vi "Convert Data.vi"(8 "error in (no error)":errorcluster, 10 "Data In":refnum<class "Data.lvclass">, 11 "Converter in":refnum<class "Converter.lvclass">) -> (0 "error out":errorcluster, 2 "Data Out":refnum<class "Data.lvclass">, 3 "Converter out":refnum<class "Converter.lvclass">)   [LabVIEW 2022 SP3, in "Converter.lvclass"]
uses:
  Converter.lvclass
  Data/Data.lvclass
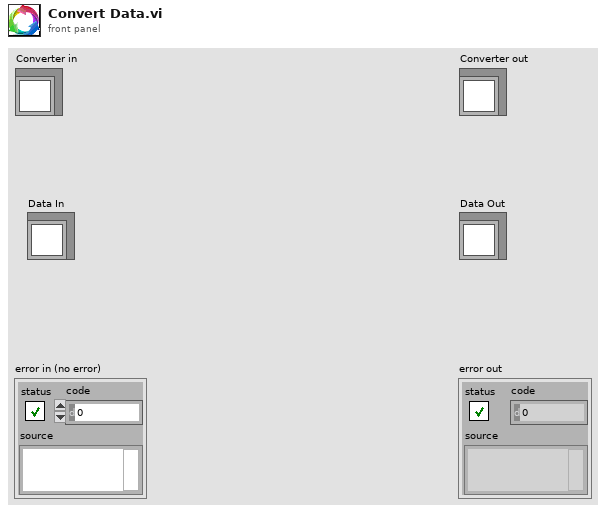
[diagram p1: front panel]
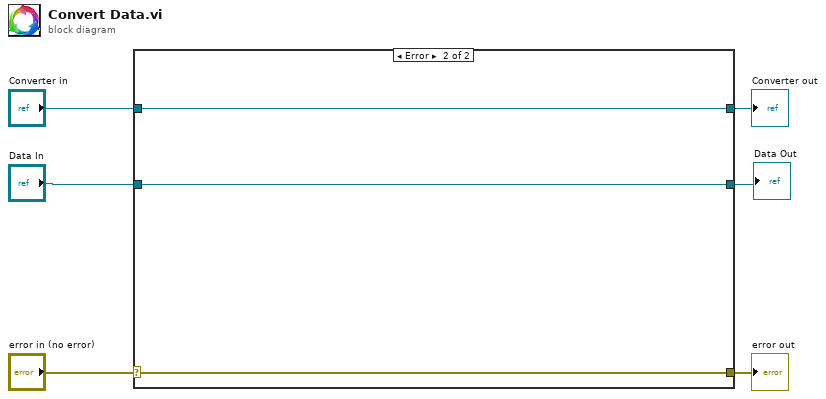
[diagram p0: block diagram]
diagram:
  n1 = case shown="Error" "error in (no error)" {
    selector: "error in (no error)" -> [w8 w12]
    tunnel: [w8 w12] -> w5
    tunnel: [w9 w11] -> w3
    tunnel: "Converter in" -> [w9 w11]
    tunnel: [w7 w10] -> w2
    tunnel: "Data In" -> [w7 w10]
    frame No Error {
      # "Wire the error cluster across even in the \"No Error\"\ncase so that warnings get propagated."
    }
    frame Error {
    }
  }
  "error out" <- w5
  "Converter out" <- w3
  "Data Out" <- w2
